vi "Flush Windows Message Queue.vi"(2 "error in (no error)":errorcluster, 3 "win msg queue":T1) -> (0 "error out":errorcluster, 1 "win msg queue out":T1)   [LabVIEW 2010, in "Windows messages for Labview (32 and 64).lvlib"]
doc: "Removes all pending windows messages in the windows message queue.\n\nParameters:\nwin msg queue: the queue whose elements should be deleted.\n\nErrors:\nReturns 6751 if win msg queue is not a valid windows message queue."
uses:
  Windows messages for Labview (32 and 64).lvlib
  Windows Messages for LabVIEW_64.dll
  Windows Messages for LabVIEW_32.dll
  Win Msg Queue RefNum.ctl
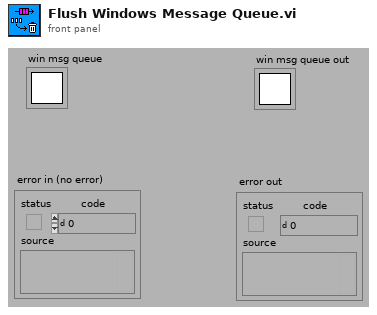
[diagram p1: front panel]
types:
  T1 = typedef "Windows messages for Labview (32 and 64).lvlib/Win Msg Queue RefNum.ctl" = refnum<k1>
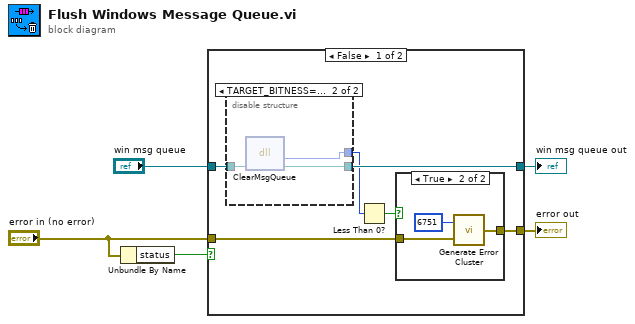
[diagram p0: block diagram]
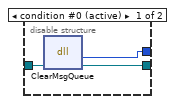
[diagram p2: hidden frame]
diagram:
  n1 = Unbundle By Name("error in (no error)") -> ("status"=w2:bool)
  n2 = case shown="False" w2 {
    tunnel: "win msg queue" -> [w8 w22]
    tunnel: "error in (no error)" -> [w11 w23]
    tunnel: [w9 w23] -> w3
    tunnel: [w7 w22] -> w1
    frame False {
      n3 = disable-structure shown="TARGET_BITNESS==32" {
        disable-tunnel: [w13 w15] -> w7
        disable-tunnel: [w12 w16] -> w6
        disable-tunnel: w8 -> [w14 w17]
        frame condition #0 (active) {
          n4 = dll-call lib="P:/hagen/PDLM/API/Demos/LabVIEW/LabVIEW2017/_lib/Windows Messages for Labview/llb/Windows Messages for LabVIEW_64.dll" fn="ClearMsgQueue"("occurrence"=w14) -> ("return type"=w12:i32, "occurrence"=w13:T1)  [unwired: 3 in, 2 out]
        }
        frame condition #1 {
          n5 = dll-call lib="D:/labview_d/temp/Windows Messaging/Windows Messages for Labview/llb/Windows Messages for LabVIEW_32.dll" fn="ClearMsgQueue"("occurrence"=w17) -> ("return type"=w16:i32, "occurrence"=w15:T1)  [unwired: 3 in, 2 out]
        }
      }
      n6 = Less Than 0?(x=w6) -> (x < 0?=w10:bool)
      n7 = case shown="True" w10 {
        tunnel: w11 -> [w18 w20]
        tunnel: [w18 w21] -> w9
        frame False {
        }
        frame True {
          n8 = call "Generate Error Cluster.vi"("error in (no error)"=w20, "Error Code"=6751) -> ("error out"=w21:errorcluster)
        }
      }
    }
    frame True {
    }
  }
  "error out" <- w3
  "win msg queue out" <- w1
